vi "Sequence Selection Dialog_Test.vi"() -> (0 "error out":errorcluster, 5 "Canceled?":bool)   [LabVIEW 2014]
uses:
  Tables/scan_array.llb/Scan Array (I32).vi
panel:
  out "subarray":string[][](array[string])
  in  "All":bool
  in  "Multicolumn Listbox":i32(listbox)
  in  "OK":bool
  in  "error in (no error)":errorcluster
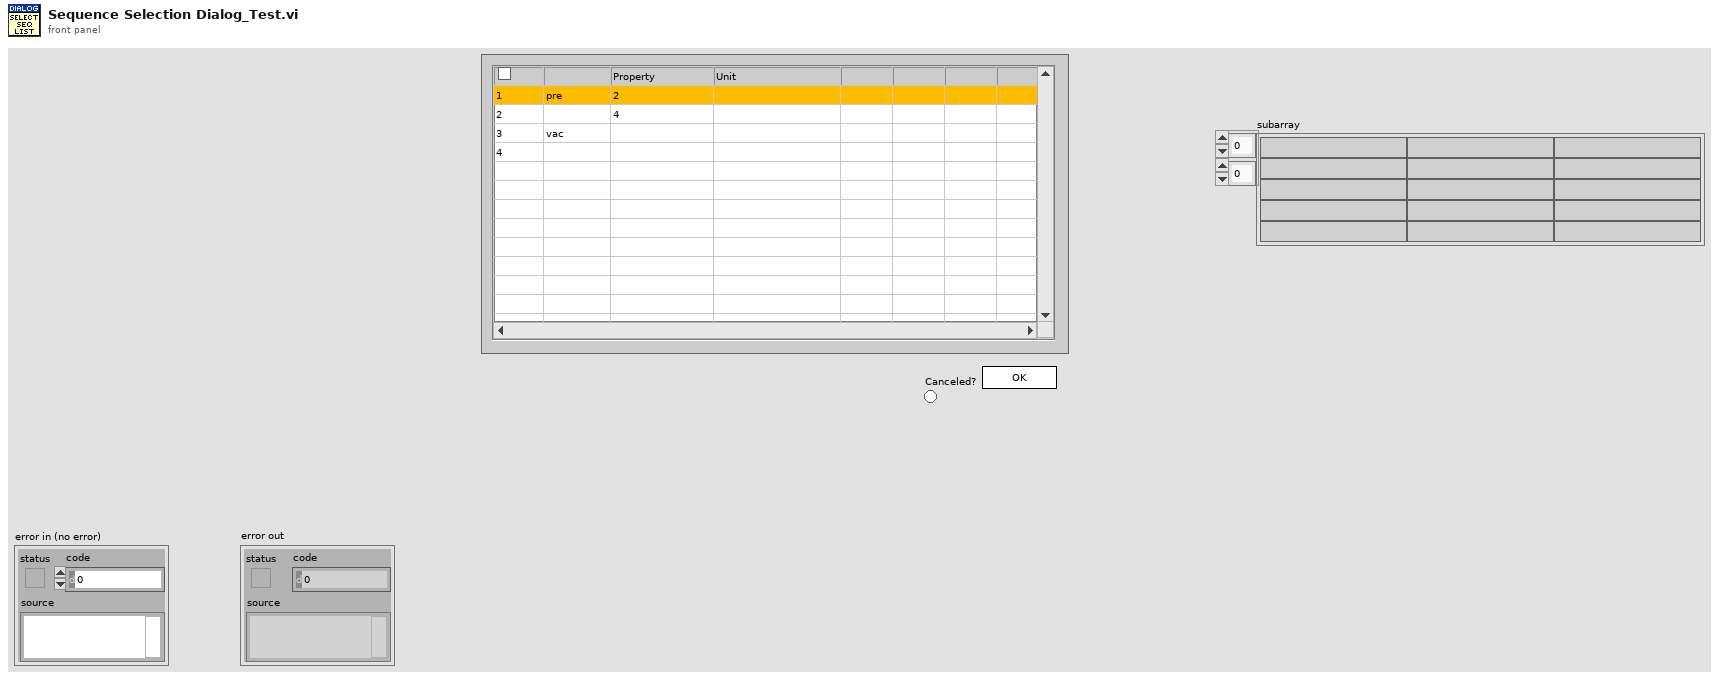
[diagram p1: front panel]
types:
  T1 = typedef "LVPoint32TypeDef.ctl" = cluster{"Horizontal":i32, "Vertical":i32}
  T2 = typedef "LVRowAndColumnTypeDef.ctl" = cluster{"Row":i32, "Column":i32}
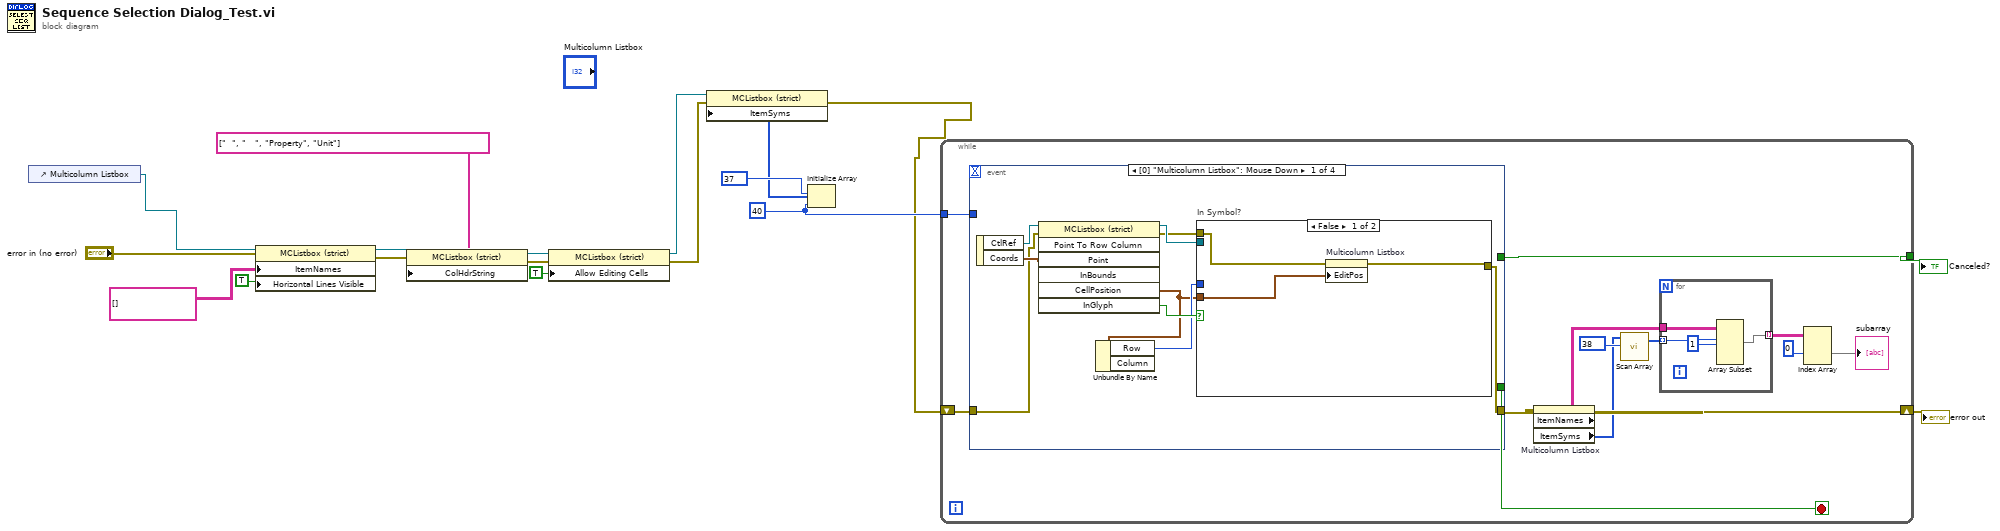
[diagram p0: block diagram]
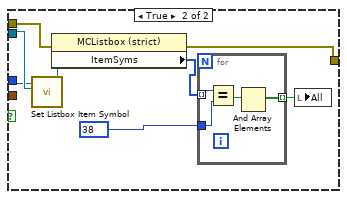
[diagram p2: hidden frame]
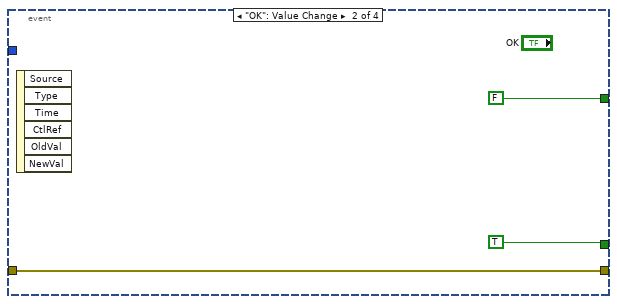
[diagram p3: hidden frame]
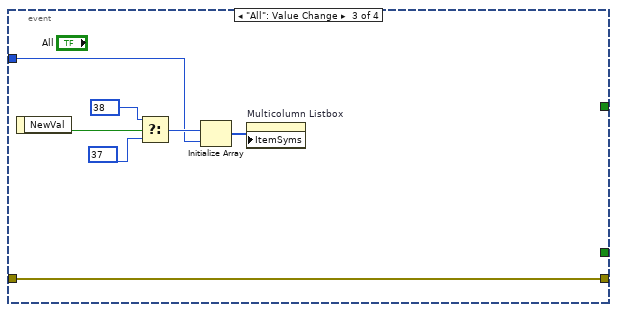
[diagram p4: hidden frame]
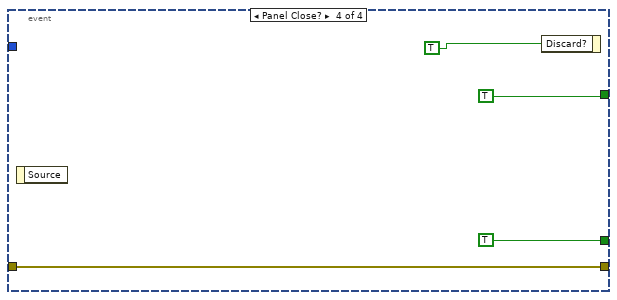
[diagram p5: hidden frame]
diagram:
  w6 = 40 ("dimension size")
  n1 = control-ref of="Multicolumn Listbox"() -> (w13:refnum<vi>)
  n2 = property class="MCListbox (strict)"(reference=w13, error in="error in (no error)", "ItemNames"=string[][] [] ("Item Names"), "Horizontal Lines Visible"=TRUE ("Visible Items:Horizontal Lines Visible")) -> (reference out=w11:refnum<vi>, error out=w12:errorcluster)
  n3 = property class="MCListbox (strict)"(reference=w11, error in=w12, "ColHdrString"=string[] ["  ", "   ", "Property", "Unit"] ("Column Header Strings[]")) -> (reference out=w10:refnum<vi>, error out=w9:errorcluster)
  n4 = property class="MCListbox (strict)"(reference=w10, error in=w9, "Allow Editing Cells"=TRUE) -> (reference out=w8:refnum<vi>, error out=w7:errorcluster)
  n5 = Initialize Array(37, w6) -> (w3:i32[])
  n6 = property class="MCListbox (strict)"(reference=w8, error in=w7, "ItemSyms"=w3) -> (error out=w1:errorcluster)  [unwired: 1 out]
  n7 = while {
    tunnel: [w24] -> w16
    tunnel: w6 -> [w22]
    shift-right: [w25] -> w17
    shift-left: w1 -> [w23]
    stop <- w21 stop-if-true
    n8 = event shown="[0] \"Multicolumn Listbox\": Mouse Down" {
      selector: _ -> [_ _ _ _]
      dyn-events: _ -> [_ _ _ _]
      timeout: _ -> [_ _ _ _]
      tunnel: w23 -> [w34 w57 w59 w68]
      tunnel: [w32 w57 w59 w68] -> w31
      tunnel: [_ TRUE ("NewVal") _ TRUE ("NewVal")] -> w21
      tunnel: [_ FALSE _ TRUE] -> w24
      tunnel: w22 -> [_ _ w61 _]
      event "Multicolumn Listbox": Mouse Down {
        n9 = event-data() -> ("CtlRef"=w40:refnum<vi>, "Coords"=w37:T1)  [unwired: 1 in]
        n10 = invoke class="MCListbox (strict)" method="Point To Row Column"(reference=w40, error in=w34, "Point"=w37) -> (reference out=w39:refnum<vi>, error out=w33:errorcluster, "CellPosition"=w35:T2, "InGlyph"=w38:bool)  [unwired: 4 in, 3 out]
        n11 = Unbundle By Name(w35) -> ("Row"=w36:i32)  [unwired: 1 out]
        n12 = case "In Symbol?" shown="False" w38 {
          tunnel: w36 -> [_ w51]
          tunnel: w39 -> [_ w52]
          tunnel: w35 -> [w43 _]
          tunnel: w33 -> [w42 w45]
          tunnel: [w41 w44] -> w32
          frame False {
            n13 = property on="Multicolumn Listbox" class="MCListbox (strict)"(error in=w42, "EditPos"=w43) -> (error out=w41:errorcluster)  [unwired: 1 in, 1 out]
          }
          frame True {
            n14 = call "Set Listbox Item Symbol.vi"("Row"=w51, "Multicolumn Listbox 2"=w52) -> ("Multicolumn Listbox 3"=w50:refnum<vi>)  [unwired: 6 in]
            n15 = property class="MCListbox (strict)"(reference=w50, error in=w45) -> (error out=w44:errorcluster, "ItemSyms"=w49:i32[])  [unwired: 1 out]
            n16 = for {
              tunnel: w49 -> [w55] mode=indexing
              tunnel: 38 -> [w54]
              tunnel: [w53] -> w47 mode=indexing
              n17 = Equal?(x=w55, y=w54) -> (x = y?=w53:bool)
            }
            n18 = And Array Elements(Boolean array=w47) -> (logical AND=w46:bool)
            n19 = local write "All"(w46) -> ()
          }
        }
      }
      event "OK": Value Change {
        n20 = event-data() -> ()  [unwired: 1 in, 6 out]
      }
      event "All": Value Change {
        n21 = event-data() -> ("NewVal"=w65:bool)  [unwired: 1 in]
        n22 = Select(t=38, s=w65, f=37) -> (s? t:f=w62:i32)
        n23 = Initialize Array(w62, w61) -> (w60:i32[])
        n24 = property on="Multicolumn Listbox" class="MCListbox (strict)"("ItemSyms"=w60) -> ()  [unwired: 2 in, 2 out]
      }
      event Panel Close? {
        n25 = event-data() -> ()  [unwired: 1 in, 1 out]
        n26 = event-data("Discard?"=TRUE) -> ()  [unwired: 1 in, 1 out]
      }
    }
    n27 = property on="Multicolumn Listbox" class="MCListbox (strict)"(error in=w31) -> (error out=w25:errorcluster, "ItemNames"=w19:string[][], "ItemSyms"=w29:i32[])  [unwired: 1 in, 1 out]
    n28 = call-poly "Scan Array.vi"("search element"=38, "Input array"=w29) -> ("Matched Indices"=w28:i32[])  [unwired: 3 in]
    n29 = for {
      tunnel: w28 -> [w73] mode=indexing
      tunnel: [w71] -> w27 mode=indexing
      tunnel: w19 -> [w70]
      n30 = Array Subset(array=w70, index (row)=w73, length (row)=1 ("length")) -> (w71:string[][])  [unwired: 2 in]
    }
    n31 = Index Array(array=w27, index (dim 1)=0 ("index (row)")) -> (element=→"subarray":string[][])  [unwired: 2 in]
  }
  "error out" <- w17
  "Canceled?" <- w16
